vi "QI_radial profile_new.vi"(11 "QI 传递变量输入":T1) -> (1 "radial profile":dbl[](array[numeric]), 2 "array R":dbl[](array[numeric]), 3 "QI 传递变量输出":T1)   [LabVIEW 2017]
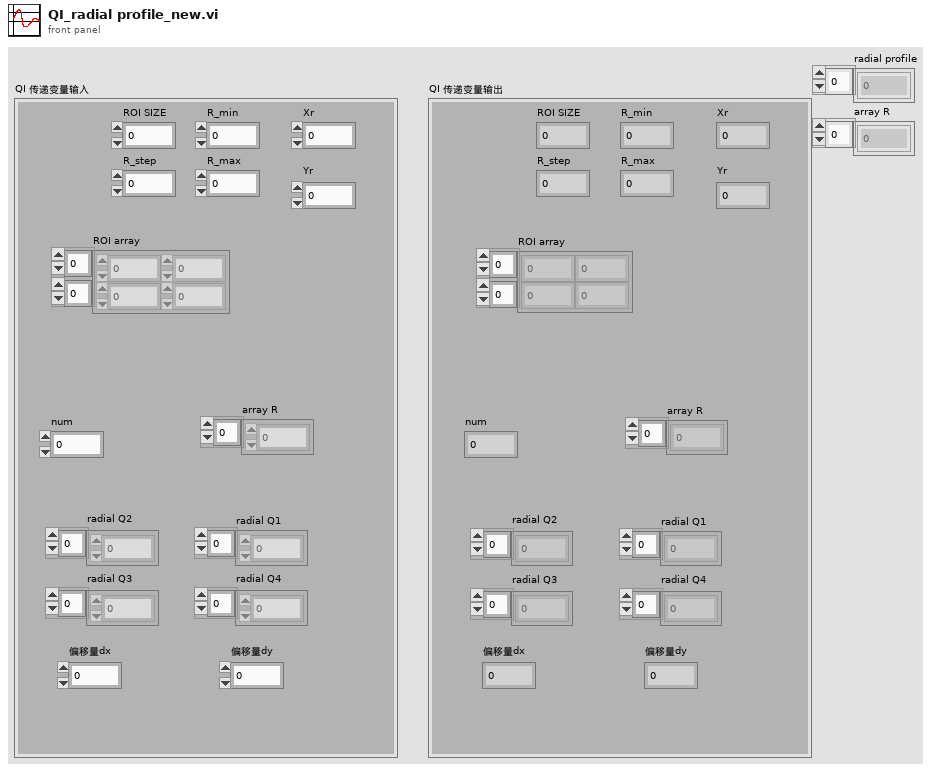
[diagram p1: front panel]
types:
  T1 = typedef "QI 传递变量.ctl" = cluster{"ROI SIZE":i32, "R_step":dbl, "R_min":dbl, "R_max":dbl, "num":dbl, "array R":dbl[], "radial Q1":dbl[], "radial Q2":dbl[], "radial Q3":dbl[], "radial Q4":dbl[], "偏移量dx":dbl, "偏移量dy":dbl, "ROI array":sgl[][], "Xr":dbl, "Yr":dbl}
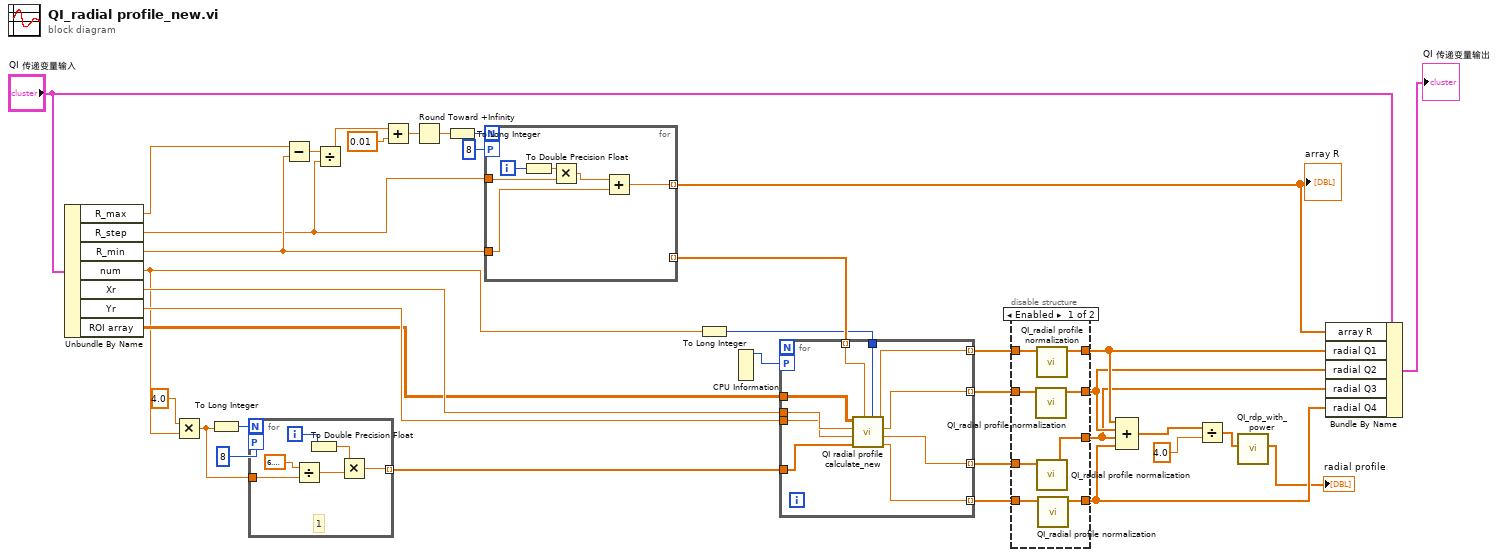
[diagram p0: block diagram]
diagram:
  n1 = Unbundle By Name("QI 传递变量输入") -> ("R_max"=w35:dbl, "R_step"=w32:dbl, "R_min"=w34:dbl, "num"=w8:dbl, "Xr"=w25:dbl, "Yr"=w24:dbl, "ROI array"=w23:sgl[][])
  n2 = Multiply(x=4.0, y=w8) -> (x*y=w9:dbl)
  n3 = To Long Integer(number=w9) -> (32bit integer=w16:i32)
  n4 = for {
    N: w16 -> [_]
    tunnel: w9 -> [w43]
    tunnel: [w39] -> w15 mode=indexing
    workers-P: 8 -> [_]
    i -> [w41]
    # "1"
    n5 = Divide(x=6.283185307179586, y=w43) -> (x/y=w42:dbl)
    n6 = To Double Precision Float(number=w41) -> (double precision float=w40:dbl)
    n7 = Multiply(x=w40, y=w42) -> (x*y=w39:dbl)
  }
  n8 = Subtract(x=w35, y=w34) -> (x-y=w33:dbl)
  n9 = Divide(x=w33, y=w32) -> (x/y=w31:dbl)
  n10 = Add(x=w31, y=0.01) -> (x+y=w29:dbl)
  n11 = Round Toward +Infinity(x=w29) -> (ceil(x): smallest int >= x=w28:dbl)
  n12 = To Long Integer(number=w28) -> (32bit integer=w27:i32)
  n13 = for "For循环" {
    N: w27 -> [_]
    tunnel: w34 -> [w46]
    tunnel: w32 -> [w48]
    tunnel: [w44] -> w22 mode=indexing
    tunnel: [w44] -> w26 mode=indexing
    workers-P: 8 -> [_]
    i -> [w49]
    n14 = To Double Precision Float(number=w49) -> (double precision float=w45:dbl)
    n15 = Multiply(x=w45, y=w48) -> (x*y=w47:dbl)
    n16 = Add(x=w47, y=w46) -> (x+y=w44:dbl)
  }
  "array R" <- w22
  n17 = To Long Integer(number=w8) -> (32bit integer=w7:i32)
  n18 = CPU Information() -> (4:w21:i32)  [unwired: 3 out]
  n19 = for "For循环" {
    tunnel: w26 -> [w57] mode=indexing
    tunnel: w25 -> [w59]
    tunnel: w24 -> [w58]
    tunnel: w23 -> [w56]
    workers-P: w21 -> [_]
    tunnel: w15 -> [w55]
    tunnel: [w54] -> w14 mode=indexing
    tunnel: [w53] -> w13 mode=indexing
    tunnel: [w52] -> w12 mode=indexing
    tunnel: [w51] -> w11 mode=indexing
    tunnel: w7 -> [w50]
    n20 = call "QI radial profile calculate_new.vi"("num"=w50, "r"=w57, "rad"=w55, "Yr"=w58, "Xr"=w59, "ROI array"=w56) -> ("mean 4"=w51:dbl, "mean 3"=w52:dbl, "mean 2"=w53:dbl, "mean"=w54:dbl)  [unwired: 2 in]
  }
  n21 = disable-structure shown="Enabled" {
    disable-tunnel: [w67 w71] -> w20
    disable-tunnel: [w66 w70] -> w19
    disable-tunnel: [w65 w69] -> w18
    disable-tunnel: [w64 w68] -> w17
    disable-tunnel: w14 -> [w63 w71]
    disable-tunnel: w13 -> [w62 w70]
    disable-tunnel: w12 -> [w61 w69]
    disable-tunnel: w11 -> [w60 w68]
    frame Enabled {
      n22 = call "QI_radial profile normalization.vi"("rp输入"=w62) -> ("rp输出"=w66:dbl[])  [unwired: 10 in]
      n23 = call "QI_radial profile normalization.vi"("rp输入"=w63) -> ("rp输出"=w67:dbl[])  [unwired: 10 in]
      n24 = call "QI_radial profile normalization.vi"("rp输入"=w61) -> ("rp输出"=w65:dbl[])  [unwired: 10 in]
      n25 = call "QI_radial profile normalization.vi"("rp输入"=w60) -> ("rp输出"=w64:dbl[])  [unwired: 10 in]
    }
    frame Disabled {
    }
  }
  n26 = Compound Arithmetic op=ADD(w20, w19, w18, w17) -> (w3:dbl[])
  n27 = Divide(x=w3, y=4.0) -> (x/y=w2:dbl[])
  n28 = call "QI_rdp_with_power.vi"("Array in"=w2) -> ("array out"=→"radial profile":dbl[])  [unwired: 10 in]
  n29 = Bundle By Name(cluster="QI 传递变量输入", "array R"=w22, "radial Q1"=w20, "radial Q2"=w19, "radial Q3"=w18, "radial Q4"=w17) -> (→"QI 传递变量输出":T1)
